vi "Cluster Make Typedef.vi"(7 "skip first typedef?":bool, 10 "Terminal in":refnum<vi>, 11 "ClusterConstant refnum in":refnum<vi>) -> (3 "String":string)   [LabVIEW 2014]
doc: "Creates Cluste C code typedefinition like:\n typedef struct {\n ...\n String ABCabc;\n int A;\n struct{int A; String B; ...;} xyzNameForStruct;\n ...\n };\n\nIf ClusterConstant refnum not wired, Terminal is used, this VI create Cluster from Terminal, observe it and remove it."
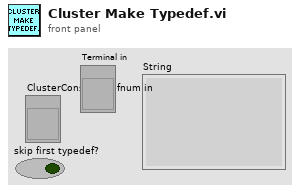
[diagram p1: front panel]
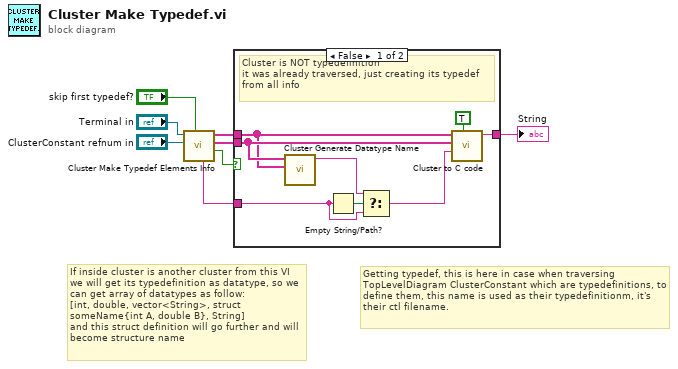
[diagram p0: block diagram]
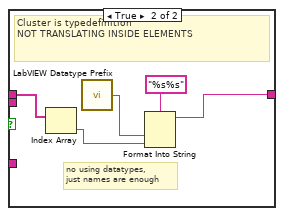
[diagram p2: hidden frame]
diagram:
  # "If inside cluster is another cluster from this VI we will get its typedefinition as datatype, so we can get array of datatypes as follow:\n[int, double, vector<String>, struct someName{int A, double B}, String]\nand this struct definition will go further and will become structure name"
  # "Getting typedef, this is here in case when traversing TopLevelDiagram ClusterConstant which are typedefinitions, to define them, this name is used as their typedefinitionm, it's their ctl filename."
  n1 = call "Cluster Make Typedef Elements Info.vi"("skip first typedef?"="skip first typedef?", "ClusterConstant refnum"="ClusterConstant refnum in", "Terminal in"="Terminal in") -> ("is typedef?"=w3:bool, "Cluster elements datatypes"=w4:string[], "Cluster elements names"=w8:string[], "typedef name"=w1:string)  [unwired: 4 in, 1 out]
  n2 = case shown="False" w3 {
    tunnel: w8 -> [w11 w18]
    tunnel: [w16 w17] -> w7
    tunnel: w4 -> [w13 _]
    tunnel: w1 -> [w14 _]
    frame False {
      # "Cluster is NOT typedefinition\nit was already traversed, just creating its typedef from all info"
      n3 = call "Cluster Generate Datatype Name.vi"("Cluster elements names"=w11, "Cluster elements datatypes"=w13) -> ("generated datatype name"=w9:string)  [unwired: 9 in]
      n4 = Empty String/Path?(string/path=w14) -> (empty?=w15:bool)
      n5 = Select(t=w9, s=w15, f=w14) -> (s? t:f=w10:string)
      n6 = call "Cluster to C code.vi"("indent code?"=TRUE, "typedef name"=w10, "Cluster elements datatypes"=w13, "Cluster elements names"=w11) -> ("C code"=w16:string)  [unwired: 7 in]
    }
    frame True {
      # "no using datatypes,\njust names are enough"
      # "Cluster is typedefinition\nNOT TRANSLATING INSIDE ELEMENTS"
      n7 = Index Array(array=w18) -> (element=w21:string)  [unwired: 1 in]
      n8 = call "LabVIEW Datatype Prefix.vi"() -> ("datatype prefix"=w20:string)
      n9 = Format Into String(format string="%s%s", w20, w21) -> (resulting string=w17:string)  [unwired: 2 in, 1 out]
    }
  }
  "String" <- w7
